vi "Configure Burnout RJC.vi"(0 "VISA resource name":refnum<visa-resource-name>, 1 "Enable External RJC (False)":bool, 2 "External RJC Value (0)":dbl min=-20000.0 max=20000.0 format="%#.1f", 5 "AI Channel (0001)":string="0001", 7 "Burnout (0 : Off)":i32(ring) items=["Off", "Up", "Down"], 11 "error in (no error)":errorcluster) -> (4 "VISA resource name out":refnum<visa-resource-name>, 6 "AI Channel":string, 15 "error out":errorcluster)   [LabVIEW 2020, in "Yokogawa GX Series.lvlib"]
doc: "Sets the burnout detection and RJC.\n\nCommands: SBurnOut, SRjc"
uses:
  <instrlib>/Yokogawa GX Series/Yokogawa GX Series.lvlib
panel:
  # "C"
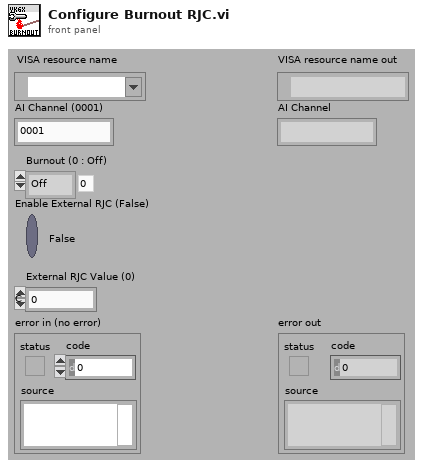
[diagram p1: front panel]
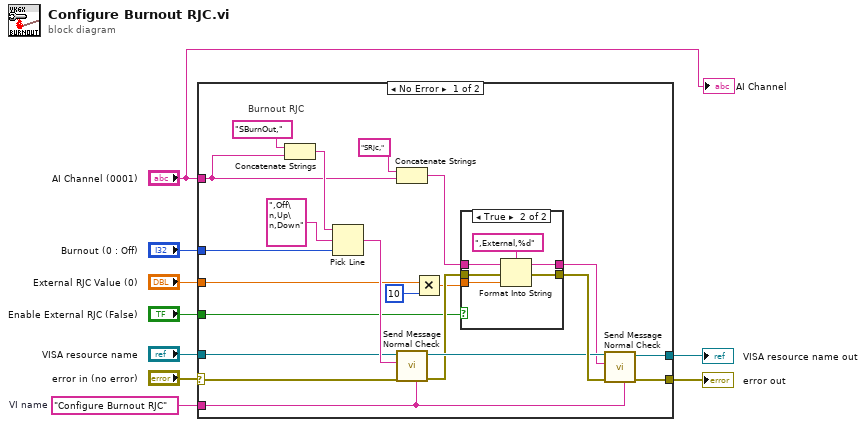
[diagram p0: block diagram]
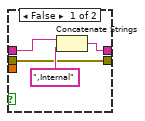
[diagram p2: hidden frame]
diagram:
  w6 = "Configure Burnout RJC"  # VI name
  n1 = case shown="No Error" "error in (no error)" {
    selector: "error in (no error)" -> [w13 w41]
    tunnel: "Burnout (0 : Off)" -> [w29 _]
    tunnel: "External RJC Value (0)" -> [w11 _]
    tunnel: "VISA resource name" -> [w23 w42]
    tunnel: w6 -> [w22 _]
    tunnel: [w19 w42] -> w5
    tunnel: [w18 w41] -> w4
    tunnel: "AI Channel (0001)" -> [w15 _]
    tunnel: "Enable External RJC (False)" -> [w14 _]
    frame No Error {
      # "Burnout RJC"
      n2 = Concatenate Strings("SBurnOut,", w15) -> (w27:string)
      n3 = Pick Line(string ("")=w27, multi-line string=",Off\n,Up\n,Down", line index=w29) -> (output string=w24:string)
      n4 = Concatenate Strings("SRjc,", w15) -> (w17:string)
      n5 = call <instrlib>:"Send Message Normal Check.vi"("Source (\"\")"=w22, "error in (no error)"=w13, "Send Message (\"\")"=w24, "VISA resource name"=w23) -> ("error out"=w20:errorcluster, "VISA resource name out"=w21:refnum<visa-resource-name>)  [unwired: 2 in, 4 out]
      n6 = Multiply(x=w11, y=10) -> (x*y=w12:dbl)
      n7 = case shown="True" w14 {
        tunnel: w12 -> [_ w39]
        tunnel: [w31 w38] -> w25
        tunnel: w20 -> [w31 w37]
        tunnel: w17 -> [w34 w36]
        tunnel: [w32 w35] -> w16
        frame False {
          n8 = Concatenate Strings(w34, ",Internal") -> (w32:string)
        }
        frame True {
          n9 = Format Into String(format string=",External,%d", initial string=w36, error in=w37, w39) -> (resulting string=w35:string, error out=w38:errorcluster)
        }
      }
      n10 = call <instrlib>:"Send Message Normal Check.vi"("Source (\"\")"=w22, "error in (no error)"=w25, "Send Message (\"\")"=w16, "VISA resource name"=w21) -> ("error out"=w18:errorcluster, "VISA resource name out"=w19:refnum<visa-resource-name>)  [unwired: 2 in, 4 out]
    }
    frame Error {
    }
  }
  "error out" <- w4
  "VISA resource name out" <- w5
  "AI Channel" <- "AI Channel (0001)"
